vi "Create New Folder.vi"() -> ()   [LabVIEW 2022 SP3]
panel:
  in  "File Name":string
  in  "Enum":enum16{"TXT", "DOC", "CSV"}(ring)
  in  "Cluster":T1
  out "error out":errorcluster
  out "Waveform Graph":dbl[](graph)
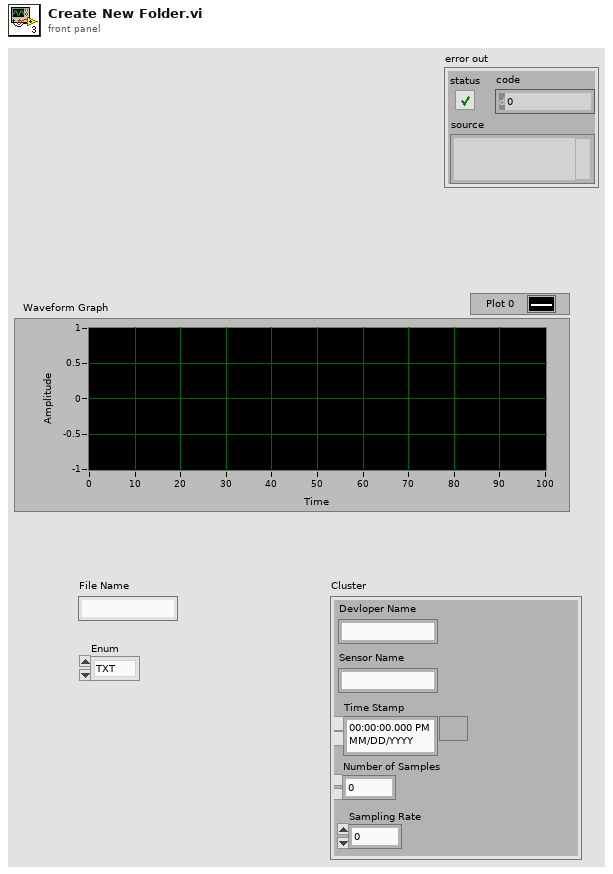
[diagram p1: front panel]
types:
  T1 = cluster{"Devloper Name ":string, "Sensor Name":string, "Time Stamp":timestamp, "Number of Samples":dbl, "Sampling Rate":dbl}
  T2 = enum16{"open", "replace", "create", "open or create", "replace or create", "replace or create with confirmation"}
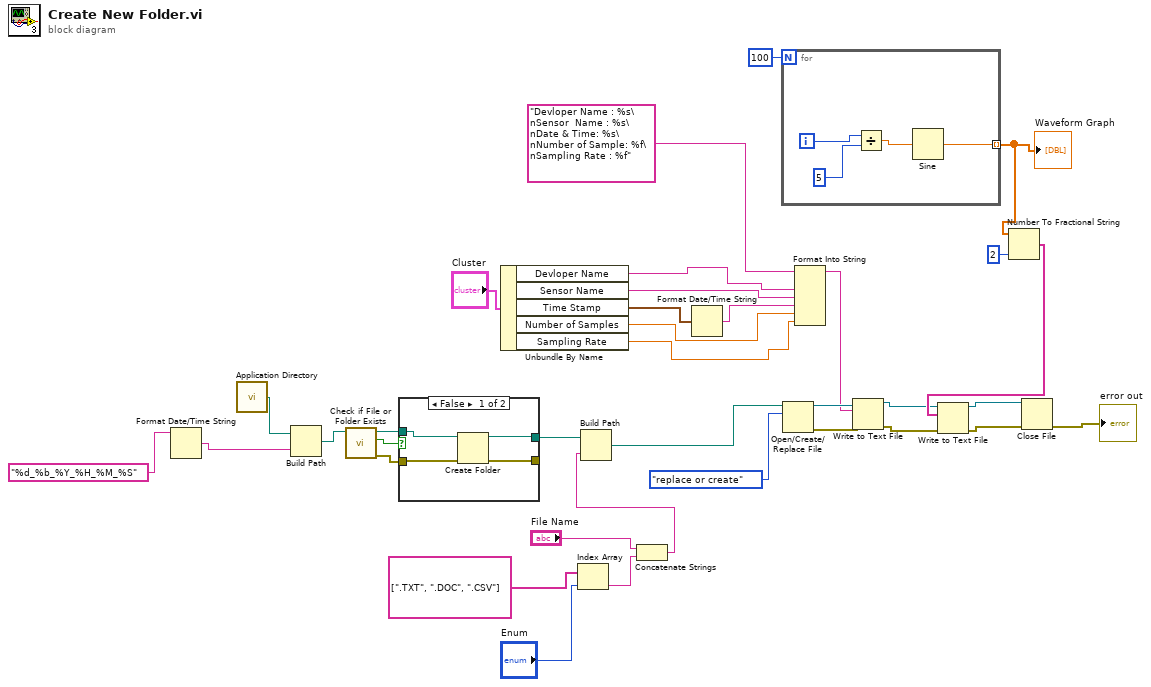
[diagram p0: block diagram]
diagram:
  n1 = Format Date/Time String(time format string (%c)="%d_%b_%Y_%H_%M_%S") -> (date/time string=w11:string)  [unwired: 2 in]
  n2 = call <vilib>:"Application Directory.vi"() -> ("Application Directory"=w13:path)
  n3 = Build Path(base path=w13, name or relative path=w11) -> (appended path=w14:path)
  n4 = call <vilib>:"Check if File or Folder Exists.vi"("path"=w14) -> ("error out"=w8:errorcluster, "file or folder exists?"=w10:bool, "dup path"=w9:path)  [unwired: 8 in]
  n5 = case shown="False" w10 {
    tunnel: [w39 w41] -> w7
    tunnel: w9 -> [w38 w41]
    tunnel: w8 -> [w37 w40]
    tunnel: [w36 w40] -> _
    frame False {
      n6 = Create Folder(path (use dialog)=w38, error in=w37) -> (created path=w39:path, error out=w36:errorcluster)  [unwired: 1 in, 1 out]
    }
    frame True {
    }
  }
  n7 = Unbundle By Name("Cluster") -> ("Devloper Name"=w19:string, "Sensor Name"=w18:string, "Time Stamp"=w17:timestamp, "Number of Samples"=w16:dbl, "Sampling Rate"=w15:dbl)
  n8 = Index Array(array=string[] [".TXT", ".DOC", ".CSV"], index="Enum") -> (element=w2:string)
  n9 = Concatenate Strings("File Name", w2) -> (w1:string)
  n10 = Build Path(base path=w7, name or relative path=w1) -> (appended path=w6:path)
  n11 = Format Date/Time String(seconds (now)=w17) -> (date/time string=w21:string)  [unwired: 2 in]
  n12 = for {
    N: 100 -> [_]
    tunnel: [w42] -> w29 mode=indexing
    i -> [w45]
    n13 = Divide(x=w45, y=5) -> (x/y=w43:dbl)
    n14 = Sine(x=w43) -> (sin(x)=w42:dbl)
  }
  "Waveform Graph" <- w29
  n15 = Open/Create/Replace File(file path (use dialog)=w6, operation (0:open)=T2."replace or create") -> (refnum out=w27:refnum<file>, error out=w26:errorcluster)  [unwired: 4 in, 1 out]
  n16 = Format Into String(format string="Devloper Name : %s\nSensor  Name : %s\nDate & Time: %s\nNumber of Sample: %f\nSampling Rate : %f", w19, w18, w21, w16, w15) -> (resulting string=w23:string)  [unwired: 2 in, 1 out]
  n17 = Write to Text File(file (use dialog)=w27, text=w23, error in=w26) -> (refnum out=w24:refnum<file>, error out=w25:errorcluster)  [unwired: 1 in, 1 out]
  n18 = Number To Fractional String(number=w29, precision (6)=i16 2) -> (F-format string=w28:string[])  [unwired: 2 in]
  n19 = Write to Text File(file (use dialog)=w24, text=w28, error in=w25) -> (refnum out=w33:refnum<file>, error out=w32:errorcluster)  [unwired: 1 in, 1 out]
  n20 = Close File(refnum=w33, error in=w32) -> (error out=→"error out":errorcluster)  [unwired: 1 out]
